vi "vi_reference_write.vi"(8 "error in (no error)":errorcluster, 10 "vi_reference":T1, 11 "interface in":refnum<class "interface.lvclass">) -> (0 "error out":errorcluster, 3 "interface out":refnum<class "interface.lvclass">)   [LabVIEW 2015, in "functional.lvlib" / "interface.lvclass"]
uses:
  interface.lvclass
  _controls/vi_reference.ctl
  interface.lvclass/interface.ctl
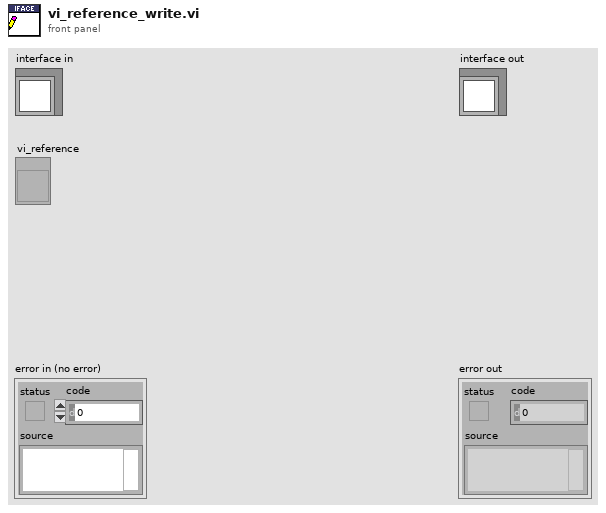
[diagram p1: front panel]
types:
  T1 = typedef "functional.lvlib/interface.lvclass/vi_reference.ctl" = refnum<vi>
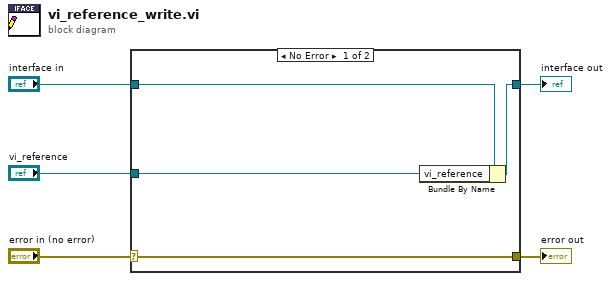
[diagram p0: block diagram]
diagram:
  n1 = case shown="No Error" "error in (no error)" {
    selector: "error in (no error)" -> [w9 w10]
    tunnel: [w9 w10] -> w4
    tunnel: [w7 w11] -> w2
    tunnel: "interface in" -> [w8 w11]
    tunnel: "vi_reference" -> [w6 _]
    frame No Error {
      n2 = Bundle By Name(cluster=w8, "vi_reference"=w6) -> (w7:refnum<class "interface.lvclass">)
    }
    frame Error {
    }
  }
  "error out" <- w4
  "interface out" <- w2
